vi "wa32 CloseHandle.vi"(8 "error in":errorcluster, 11 "handle":i32) -> (0 "error out":errorcluster)   [LabVIEW 2020, in "GOLPI library.lvlib"]
doc: "WinAPI CloseHandle() wrapper. Closes any Windoze handle. Ignores input error, but can generate error."
uses:
  <vilib>/Utility/error.llb/Error Cluster From Error Code.vi
  <vilib>/ErrorRing/Error Ring.xnode
  GOLPI library.lvlib
  kernel32.dll
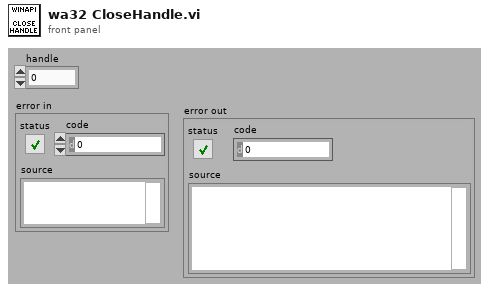
[diagram p1: front panel]
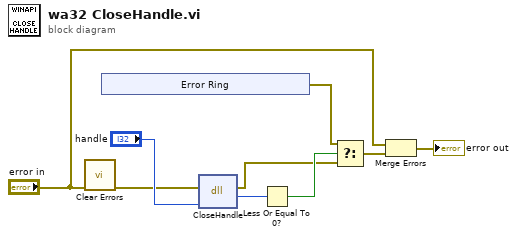
[diagram p0: block diagram]
diagram:
  n1 = call <vilib>:"Clear Errors.vi"("error in (no error)"="error in") -> ("error out"=w4:errorcluster)  [unwired: 5 in, 1 out]
  n2 = xnode "Error Ring"() -> ("error out"=w6:errorcluster)
  n3 = dll-call lib="kernel32.dll" fn="CloseHandle"(error in=w4, "handle"="handle") -> (error out=w7:errorcluster, "errout"=w9:i32)  [unwired: 3 in, 1 out]
  n4 = Less Or Equal To 0?(x=w9) -> (x <= 0?=w8:bool)
  n5 = Select(t=w6, s=w8, f=w7) -> (s? t:f=w3:errorcluster)
  n6 = Merge Errors("error in", w3) -> (→"error out":errorcluster)
